vi "Dashboard Main.vi"() -> ()   [LabVIEW 2014]
uses:
  <vilib>/event_ctls.llb/eventvkey.ctl
  <vilib>/Rock Robotics/WPI/Dashboard/WPI_DashboardLogging Global.vi
  <vilib>/Rock Robotics/Network Tables/SD Read Number.vi
  <vilib>/Rock Robotics/Network Tables/SD Write Number.vi
  <vilib>/Utility/config.llb/Write Key (String).vi
  <vilib>/Utility/config.llb/Write Key (I32).vi
  <vilib>/Utility/config.llb/NI_LVConfig.lvlib
panel:
  in  "angle":dbl(slide) scale=0.0..360.0
  in  "kD":dbl
  in  "kI":dbl
  in  "kP":dbl
  out "PID Chart":T1(graph)
  in  "TCP":refnum<k5>
  in  "Rec Mode":enum32{"Stop", "Record", "Playback"}(radio)
  in  "Vision":u16(ring) items=["Camera Off", "USB Camera SW", "USB Camera HW", "IP Camera"]
  out "Camera IP":string
  out "Image Message":string="Timeout in Camera Communications"
  in  "Dashboard Tab":T2(tab)
  in  "Camera Settings":T3={"Frame Rate"=30, "Compression"=30, "Size"=1} {"Frame Rate" scale=1.0..30.0; "Size" items=["640x480", "320x240", "160x120"]}
  out "MotorChart R":cluster{"Numeric":dbl, "Numeric":dbl}(graph)
  out "MotorChart L":T4(graph)
  out "MotorSliders R":cluster{"MotorSlide1":dbl, "MotorSlide2":dbl} {"MotorSlide2" scale=-1.0..1.0 scale format="%#_2e"; "MotorSlide1" scale=-1.0..1.0 scale format="%#_2e"}
  out "MotorSliders L":T5 {"MotorSlide4 2" scale=0.0..14.0 scale format="%#_2e"; "MotorSlide2" scale=-1.0..1.0 scale format="%#_2e"; "MotorSlide1" scale=-1.0..1.0 scale format="%#_2e"}
  out "Gyro":dbl(knob) scale=0.0..360.0
  out "JS1 Z":dbl(slide) scale=-1.0..1.0 scale format="%#_2e"
  out "JS1 Graph":cluster{"X":dbl, "Y":dbl}[](graph)
  out "JS1 Buttons":T6
  out "JS2 Z":dbl(slide) scale=-1.0..1.0 scale format="%#_2e"
  out "JS2 Graph":cluster{"X":dbl, "Y":dbl}[](graph)
  out "JS2 Buttons":T6
  out "Mode":T7(ring)=enum."Auto Disabled"
  in  "DB Camera Config":bool
  out "fps":dbl format="%#.1g"
  out "Mbps":dbl format="%#.1g"
  out "Mbps 2":bool
  in  "DB/String 9":string
  in  "DB/String 8":string
  in  "DB/String 7":string
  in  "DB/String 6":string
  in  "DB/String 5":string
  in  "DB/String 4":string
  in  "DB/String 3":string
  in  "DB/String 2":string
  in  "DB/String 1":string
  in  "DB/String 0":string
  in  "DB/Slider 0":dbl(slide) scale=0.0..5.0
  in  "DB/Slider 1":dbl(slide) scale=0.0..5.0
  in  "DB/Slider 2":dbl(slide) scale=0.0..5.0
  in  "DB/Slider 3":dbl(slide) scale=0.0..5.0
  out "DB/LED 3":bool
  out "DB/LED 2":bool
  out "DB/LED 1":bool
  out "DB/LED 0":bool
  in  "DB/Button 3":bool
  in  "DB/Button 2":bool
  in  "DB/Button 1":bool
  in  "DB/Button 0":bool caption="New Name"
  in  "Test Slider":dbl(slide) scale=0.0..100.0 scale format="%#_3g"
  in  "On/Off":bool caption="Solenoid"
  in  "Test Name":u16(ring) items=["Select the test to run...", "Example Test", "-------------------------------", "List of tests is built in robot code.", "Replace with your own automated tests."]
  in  "Test Tree":string(tree)
  in  "Motor":cluster{"Value":dbl, "Enable":bool} {"Value" scale=-1.0..1.0 scale format="%#_3g"}
  out "Progress":T8 {"Test Progress" scale=0.0..100.0}
  in  "Rev/Fwd":cluster{"Forward":bool, "Reverse":bool}
  in  "Test Ring":u16(ring) items=["Monochrome", "Color"]
  in  "Listbox":i32(listbox)
  out "Tree":string(tree)
  out "Camera Image":T9(plugin-control)
  out "Boolean":bool
  # "Left"
  # "Front"
  # "Right"
  # "Battery"
  # "This tab is a great place for autonomous settings and robot-specific values.\nPlace controls and indicators inside this tab and match name to\nDashboard Variables on robot. You can also delete this comment."
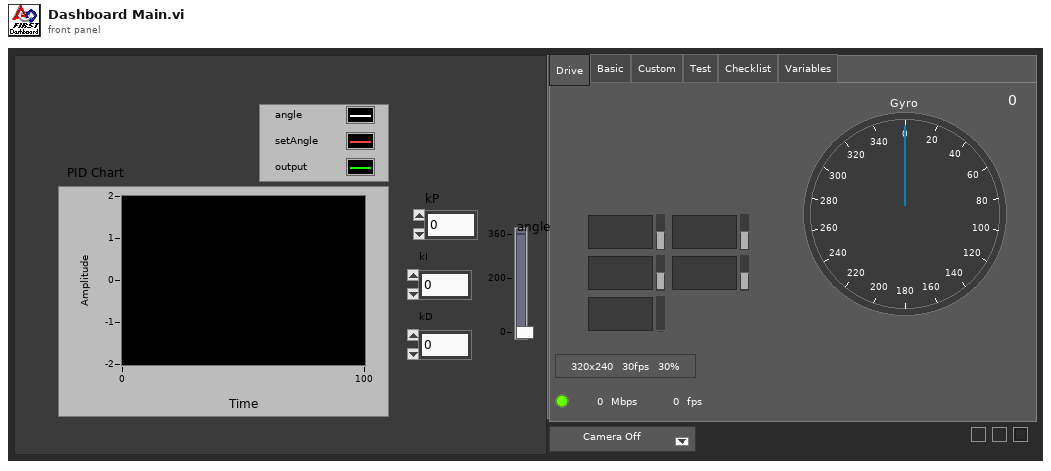
[diagram p1: front panel]
types:
  T1 = cluster{"Numeric":dbl, "Numeric":dbl, "Numeric":dbl}
  T2 = enum32{"Drive", "Basic", "Custom", "Test", "Checklist", "Variables"}
  T3 = cluster{"Frame Rate":i32, "Compression":i32, "Size":u16}
  T4 = cluster{"Numeric":dbl, "Numeric":dbl, "Battery V":dbl}
  T5 = cluster{"MotorSlide1":dbl, "MotorSlide2":dbl, "MotorSlide4 2":dbl}
  T6 = cluster{bool, bool, bool, bool, bool, bool, bool, bool, bool, bool, bool, bool}
  T7 = enum8{"Tele-Op Disabled", "Tele-Op Enabled", "Auto Disabled", "Auto Enabled", "Test Disabled", "Test Enabled", "Disconnected", "No Code", "E-Stop"}
  T8 = cluster{"Test Progress":u8, "Test Progress Text":string}
  T9 = typedef "IMAQ Image.ctl" = refnum<image>
  T10 = typedef "Image Type" = u32
  T11 = cluster{"Camera Image":refnum<vi>, "Dashboard Tab":refnum<vi>, "Boolean":refnum<vi>, "Vision":refnum<vi>, "Rec Mode":refnum<vi>, "Test Slider":refnum<vi>, "On/Off ":refnum<vi>, "Test Ring":refnum<vi>, "Rev/Fwd":refnum<vi>, "Test Name":refnum<vi>, "Motor":refnum<vi>, "Progress":refnum<vi>, "CheckList":refnum<vi>, "Tree":refnum<vi>, "Test Tree":refnum<vi>}
  T12 = cluster{"Error Strings":string, "Disable Counts":cluster{u16, u16}, "Rail Faults":cluster{u16, u16, u16}, "Robot IP":string, "DB Mode":u8, "Event Info":cluster{"Name":string, "Type":u8, "Number":u16, "Replay":u8}, "Camera Addr":string}
  T13 = cluster{"Storage":cluster{"Disk Free":u64, "RAM Block":u32, "RAM free":u32}, "CPU Utilization":cluster{"CPU % ISR":sgl, "CPU % Time Crit":sgl, "CPU % Timed Str":sgl, "CPU % High":sgl, "CPU % Above":sgl, "CPU % Normal":sgl, "CPU % Low":sgl}, "CAN":cluster{"% Bus Utilization":sgl, "Bus Off Cnt":u32, "TX_FIFO Full Cnt":u32, "Receive Error Cnt":u8, "Transmit Error Cnt":u8}, "HID":cluster{"HID Outputs":u32, "Rumble Low":u16, "Rumble High":u16}[]}
  T14 = cluster{"Status bits":cluster{"Test Mode":bool, "Autonomous":bool, "Enabled":bool, "Code Start":bool, "Brownout":bool, "Reserved 2":bool, "Reserved 3":bool, "E-Stop":bool}, "Code Trace":cluster{"Disabled":bool, "TeleOp":bool, "Auto":bool, "Test":bool}, "Controller Type":enum16{"unknown", "cRIO", "roboRio"}, "Code?":enum16{"unknown", "noCode", "code"}, "Battery V":dbl}
  T15 = cluster{"Control Bits":cluster{"TestMode":bool, "Autonomous":bool, "Enabled":bool, "FMS Present":bool, bool, bool, bool, "E-Stop":bool}, "Team Station ":u8, "Countdown":sgl, "Joystick Values":cluster{"Axes":dbl[], "Buttons":bool[], "POVs":i16[]}[]}
  T16 = cluster{"Axes":dbl[], "Buttons":bool[], "POVs":i16[]}[]
  T17 = cluster{"Axes":dbl[], "Buttons":bool[], "POVs":i16[]}
  T18 = cluster{"Buttons[0]":bool, "Buttons[1]":bool, "Buttons[2]":bool, "Buttons[3]":bool, "Buttons[4]":bool, "Buttons[5]":bool, "Buttons[6]":bool, "Buttons[7]":bool, "Buttons[8]":bool, "Buttons[9]":bool, "Buttons[10]":bool, "Buttons[11]":bool}
  T19 = typedef "NI_LVConfig.lvlib/Config Data RefNum.ctl" = refnum<k1>
  T20 = cluster{"Operation":enum16{"Update", "Clear"}, "Color Box":u32}[]
  T21 = typedef "eventvkey.ctl" = enum16{"ASCII", "Enter", "Return", "Shift", "Ctrl", "Alt", "Cmd", "Opt", "Caps", "NumLock", "Clear", "Break", "Up", "Down", "Left", "Right", "Insert", "Delete", "Home", "End", "PageUp", "PageDown", "Escape", "Help", "Pause", "ScrollLock", "F1", "F2", "F3", "F4", "F5", "F6", "F7", "F8", "F9", "F10", "F11", "F12", "F13", "F14", "F15", "F16", "F17", "F18", "F19", "F20", "F21", "F22", "F23", "F24", "Play", "VolumeUp", "VolumeDown", "Mute", "Two Byte Char"}
  T22 = cluster{"Image Size":bool, "Image Type":bool, "Pixel Value":bool, "ROI Information":bool, "Zoom Factor":bool}
  T23 = enum8{"Enabled", "Disabled", "Disabled and Grayed Out"}
  T24 = cluster{"Operation":enum16{"Update", "Clear"}, "Color Box":u32}
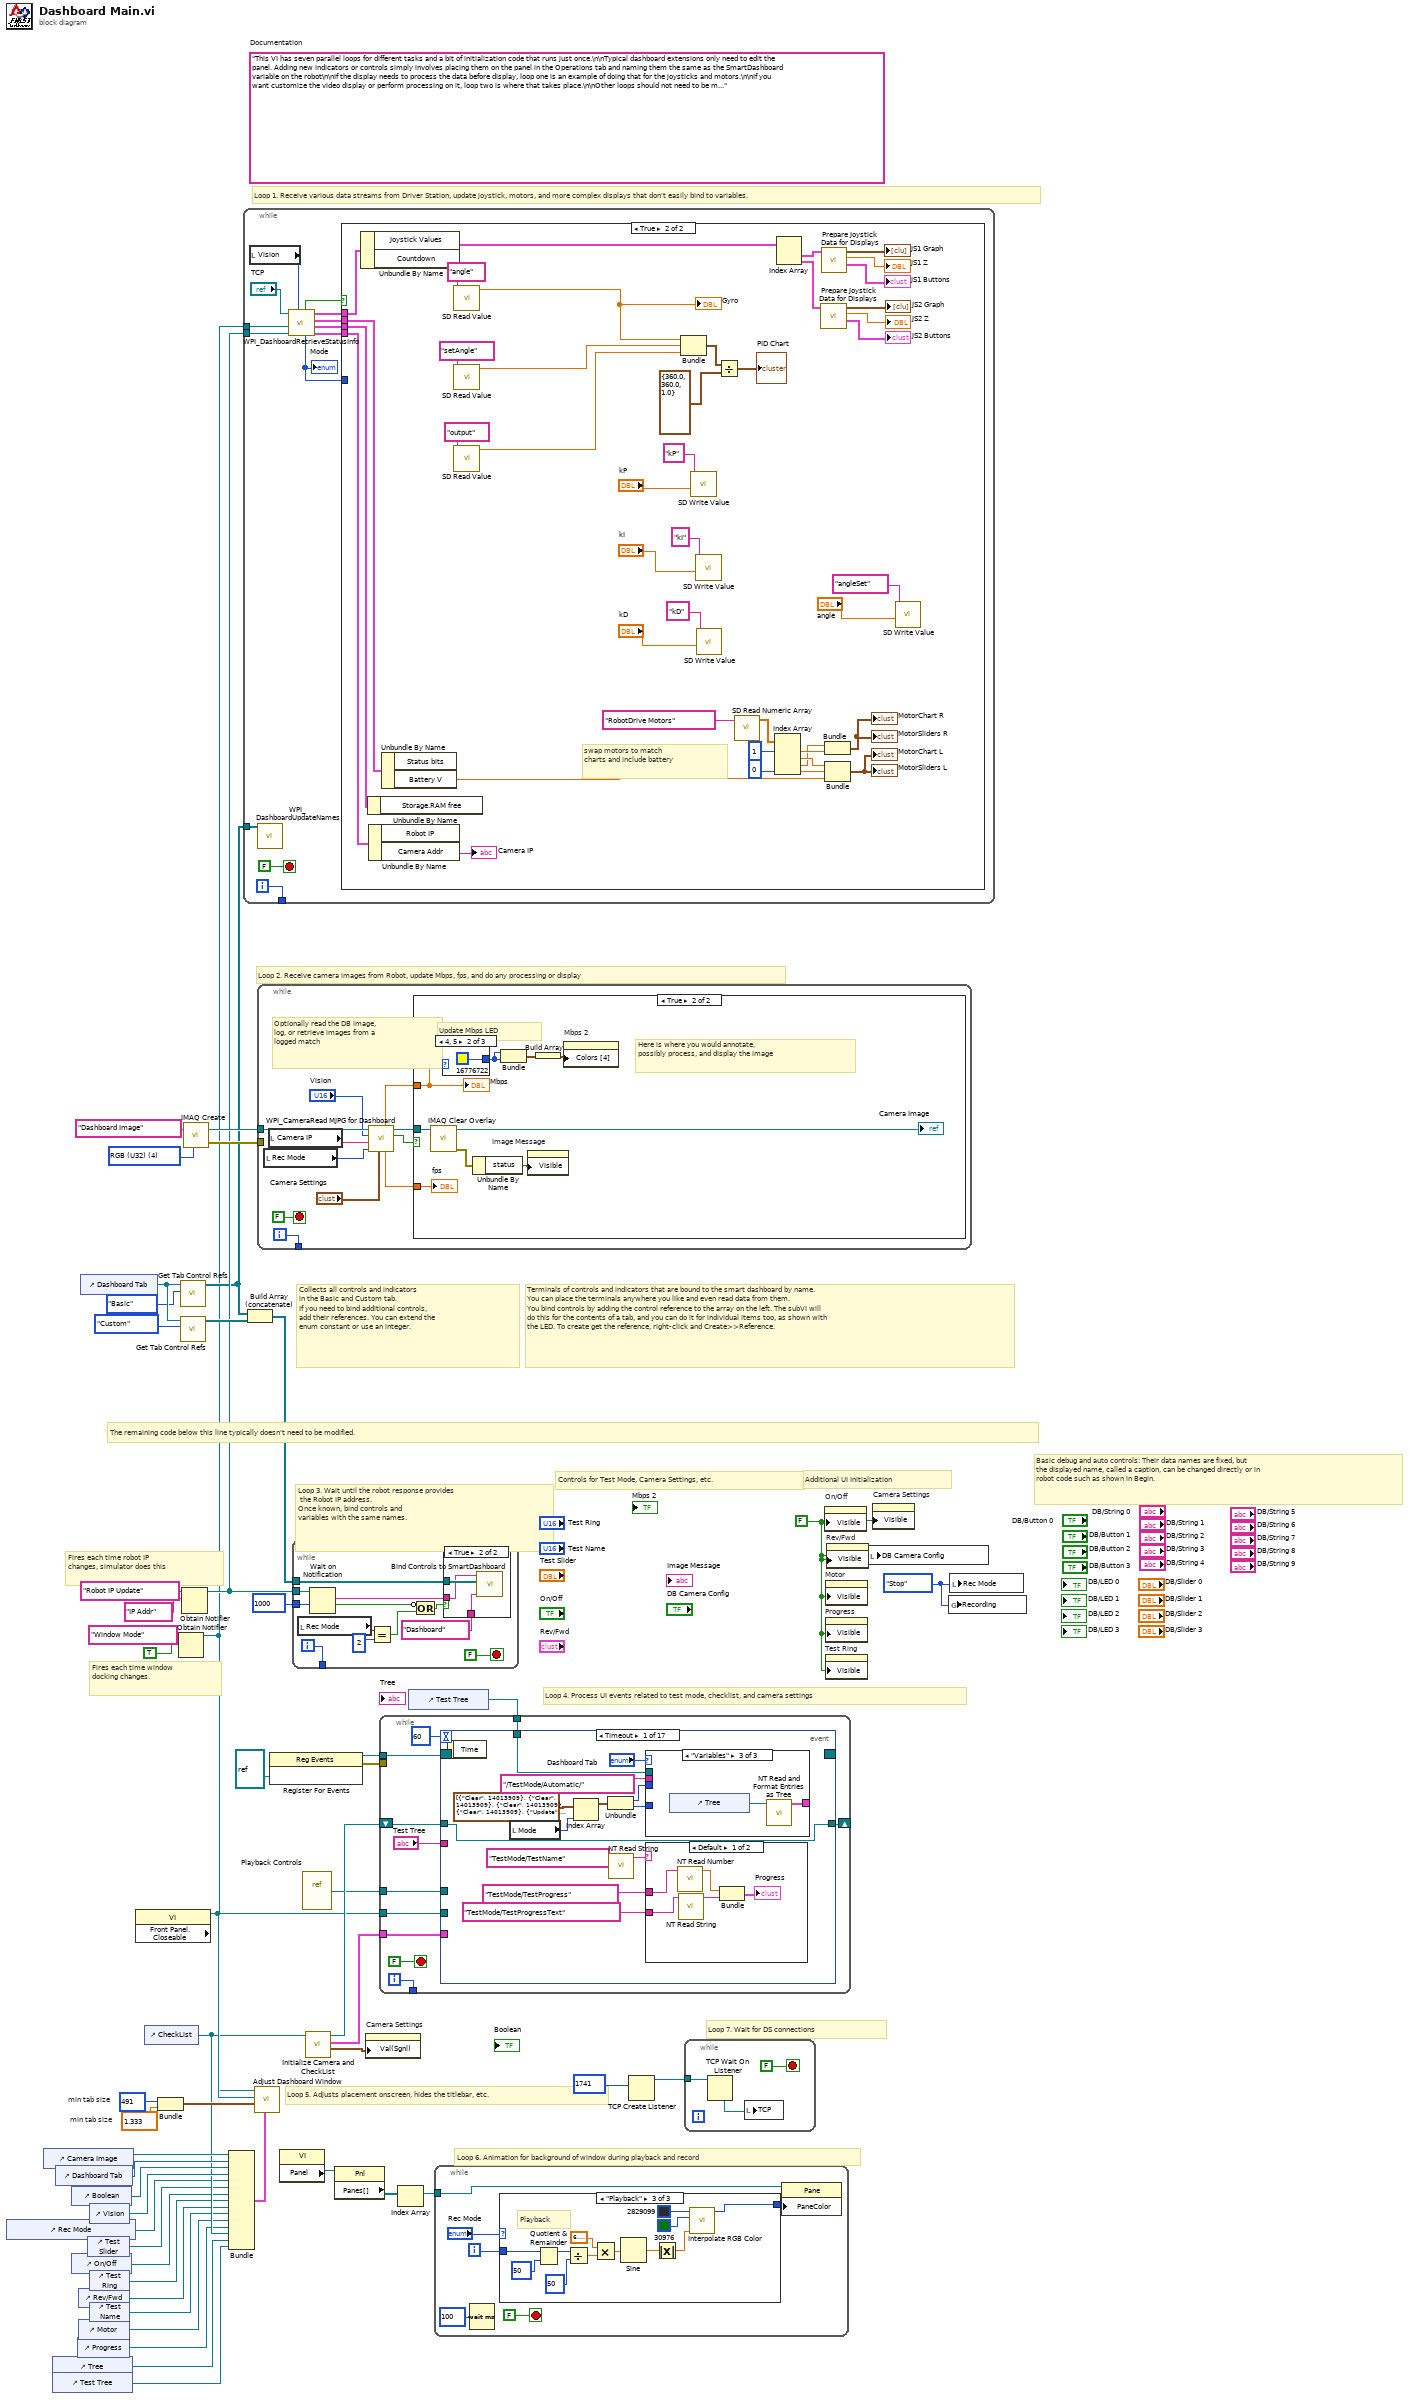
[diagram p0: block diagram]
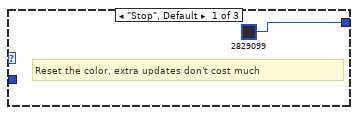
[diagram p3: hidden frame]
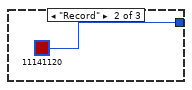
[diagram p4: hidden frame]
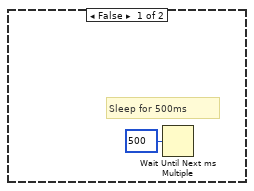
[diagram p6: hidden frame]
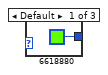
[diagram p7: hidden frame]
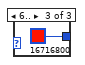
[diagram p8: hidden frame]
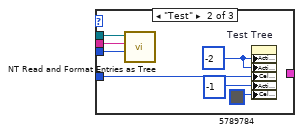
[diagram p10: hidden frame]
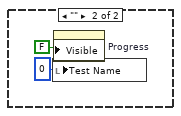
[diagram p11: hidden frame]
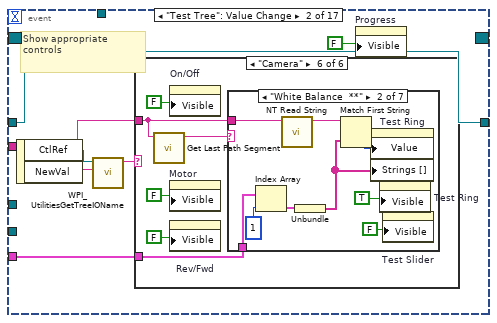
[diagram p12: hidden frame]
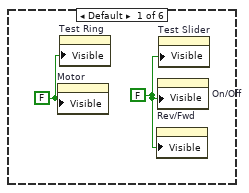
[diagram p13: hidden frame]
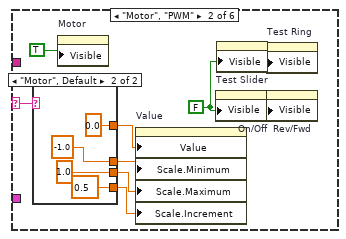
[diagram p14: hidden frame]
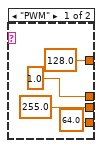
[diagram p15: hidden frame]
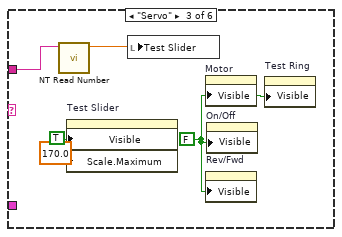
[diagram p16: hidden frame]
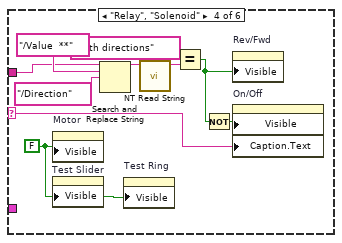
[diagram p17: hidden frame]
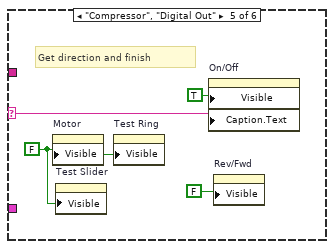
[diagram p18: hidden frame]
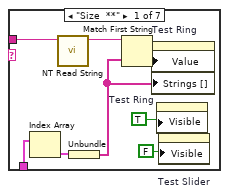
[diagram p19: hidden frame]
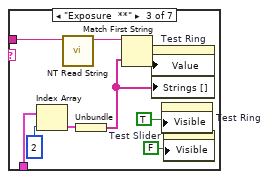
[diagram p20: hidden frame]
diagram:
  w24 = 491  # min tab size
  w23 = 1.333  # min tab size
  w32 = enum32{"Stop", "Record", "Playback"}."Stop" ("Rec Mode")
  w6 = FALSE ("Visible")
  (unwired) "This VI has seven parallel loops for different tasks and a bit of initialization code that runs just once.\n\nTypical dashboard extensions only need to edit the panel. Adding new indicators or controls simply involves placing them on the panel in the Operations tab and naming them the same as the SmartDashboard variable on the robot\n\nIf the display needs to process the data before display, loop one is an example of doing that for the joysticks and motors.\n\nIf you want customize the video display or perform processing on it, loop two is where that takes place.\n\nOther loops should not need to be modified. They are pretty standard, and document the task they perform."  # Documentation
  w52 = T10 4 items=["Grayscale (U8)", "Grayscale (I16)", "Grayscale (SGL)", "Complex (CSG)", "RGB (U32)", "HSL (U32)", "RGB (U64)"] ("Image Type")
  # "Loop 7. Wait for DS connections"
  # "Basic debug and auto controls: Their data names are fixed, but\nthe displayed name, called a caption, can be changed directly or in\nrobot code such as shown in Begin."
  # "Controls for Test Mode, Camera Settings, etc."
  # "Additional UI Initialization"
  # "Loop 6. Animation for background of window during playback and record"
  # "Fires each time robot IP\nchanges, simulator does this"
  # "Fires each time window\ndocking changes."
  # "Collects all controls and indicators\nin the Basic and Custom tab.\nIf you need to bind additional controls,\nadd their references. You can extend the\nenum constant or use an integer."
  # "The remaining code below this line typically doesn't need to be modified."
  # "Loop 4. Process UI events related to test mode, checklist, and camera settings"
  # "Terminals of controls and indicators that are bound to the smart dashboard by name.\nYou can place the terminals anywhere you like and even read data from them.\nYou bind controls by adding the control reference to the array on the left. The subVI will\ndo this for the contents of a tab, and you can do it for individual items too, as shown with\nthe LED. To create get the reference, right-click and Create>>Reference."
  # "Loop 3. Wait until the robot response provides\n the Robot IP address.\nOnce known, bind controls and\nvariables with the same names."
  # "Loop 5. Adjusts placement onscreen, hides the titlebar, etc."
  # "Loop 1. Receive various data streams from Driver Station, update joystick, motors, and more complex displays that don't easily bind to variables."
  # "Loop 2. Receive camera images from Robot, update Mbps, fps, and do any processing or display"
  n1 = control-ref of="Rec Mode"() -> (w12:refnum<vi>)
  n2 = control-ref of="Camera Image"() -> (w27:refnum<vi>)
  n3 = control-ref of="Tree"() -> (w16:refnum<vi>)
  n4 = control-ref of="Test Tree"() -> (w15:refnum<vi>)
  n5 = control-ref of="Dashboard Tab"() -> (w26:refnum<vi>)
  n6 = control-ref of="Boolean"() -> (w21:refnum<vi>)
  n7 = control-ref of="On/Off"() -> (w10:refnum<vi>)
  n8 = control-ref of="Progress"() -> (w7:refnum<vi>)
  n9 = control-ref of="Rev/Fwd"() -> (w8:refnum<vi>)
  n10 = control-ref of="Motor"() -> (w13:refnum<vi>)
  n11 = control-ref of="Dashboard Tab"() -> (w30:refnum<vi>)
  n12 = control-ref of="Test Slider"() -> (w11:refnum<vi>)
  n13 = control-ref of="Vision"() -> (w25:refnum<vi>)
  n14 = control-ref of="Test Ring"() -> (w9:refnum<vi>)
  n15 = control-ref of="Test Name"() -> (w14:refnum<vi>)
  n16 = property class="VI" props=["Front Panel.Closeable"]() -> (reference out=w31:refnum<vi>)  [unwired: 2 in, 2 out]
  n17 = control-ref of="CheckList"() -> (w17:refnum<vi>)
  n18 = Bundle("min tab size"=w24, "min tab size"=w23) -> (w22:cluster{"min tab size":i32, "min tab size":dbl})  [unwired: 1 in]
  n19 = Obtain Notifier(name (unnamed)="Window Mode", notification data type=TRUE) -> (notifier out=w3:refnum<notifier>)  [unwired: 2 in, 2 out]
  n20 = call <vilib>:"Get Tab Control Refs.vi"("Page Index"=T2."Basic" ("Dashboard Tab"), "TabControl in"=w30) -> ("ControlsOnPage"=w4:refnum<vi>[])  [unwired: 9 in]
  n21 = call <vilib>:"Get Tab Control Refs.vi"("Page Index"=T2."Custom" ("Dashboard Tab"), "TabControl in"=w30) -> ("ControlsOnPage"=w29:refnum<vi>[])  [unwired: 9 in]
  n22 = Obtain Notifier(name (unnamed)="Robot IP Update", notification data type="IP Addr" ("name (unnamed)")) -> (notifier out=w5:refnum<notifier>)  [unwired: 2 in, 2 out]
  n23 = call "IMAQ Create"("Image Name"="Dashboard Image", "Image Type"=w52) -> ("New Image"=w50:T9, "error out"=w49:errorcluster)  [unwired: 2 in, 1 out]
  n24 = Bundle("Camera Image"=w27, "Dashboard Tab"=w26, "Boolean"=w21, "Vision"=w25, "Rec Mode"=w12, "Test Slider"=w11, "On/Off"=w10, "Test Ring"=w9, "Rev/Fwd"=w8, "Test Name"=w14, "Motor"=w13, "Progress"=w7, "CheckList"=w17, "Tree"=w16, "Test Tree"=w15) -> (w18:T11)  [unwired: 1 in]
  n25 = while {
    tunnel: [w64] -> _
    tunnel: w5 -> [w58]
    tunnel: w4 -> [w57]
    tunnel: w3 -> [w53]
    i -> [w64]
    stop <- FALSE stop-if-true
    n26 = local read "Vision"() -> (w55:u16)
    n27 = call <vilib>:"WPI_DashboardUpdateNames.vi"("Controls on Tab"=w57) -> ()  [unwired: 11 in]
    n28 = call <vilib>:"WPI_DashboardRetrieveStatusInfo.vi"("Vision"=w55, "Binding Refnum"=w58, "Window Mode Notifier"=w53, "TCP Cnx"="TCP") -> ("Power and Errors"=w59:T12, "Robot Metrics"=w62:T13, "Status Info"=w63:T14, "Control Info"=w60:T15, "Robot Mode"=w56:T7, "Process?"=w61:bool)  [unwired: 2 in]
    "Mode" <- w56
    n29 = case shown="True" w61 {
      tunnel: w63 -> [_ w107]
      tunnel: w62 -> [_ w106]
      tunnel: w60 -> [_ w105]
      tunnel: w59 -> [_ w104]
      tunnel: w56 -> [_ _]
      frame False {
      }
      frame True {
        # "swap motors to match\ncharts and include battery"
        n30 = Unbundle By Name(w105) -> ("Joystick Values"=w92:T16)  [unwired: 1 out]
        n31 = Unbundle By Name(w106) -> ()  [unwired: 1 out]
        n32 = Unbundle By Name(w104) -> ("Camera Addr"=→"Camera IP":string)  [unwired: 1 out]
        n33 = Unbundle By Name(w107) -> ("Battery V"=w93:dbl)  [unwired: 1 out]
        n34 = call-poly <vilib>:"SD Read Value.vi"("Name"="angle") -> ("Numeric"=w68:dbl)  [unwired: 8 in, 2 out]
        "Gyro" <- w68
        n35 = call-poly <vilib>:"SD Read Value.vi"("Name"="setAngle") -> ("Numeric"=w80:dbl)  [unwired: 8 in, 2 out]
        n36 = call-poly <vilib>:"SD Read Value.vi"("Name"="output") -> ("Numeric"=w78:dbl)  [unwired: 8 in, 2 out]
        n37 = Bundle("Numeric"=w68, "Numeric"=w80, "Numeric"=w78) -> (w76:T1)  [unwired: 1 in]
        n38 = call-poly <vilib>:"SD Write Value.vi"("Numeric"="kP", "Name"="kP") -> ()  [unwired: 8 in, 2 out]
        n39 = call-poly <vilib>:"SD Write Value.vi"("Numeric"="kI", "Name"="kI") -> ()  [unwired: 8 in, 2 out]
        n40 = call-poly <vilib>:"SD Write Value.vi"("Numeric"="kD", "Name"="kD") -> ()  [unwired: 8 in, 2 out]
        n41 = Divide(x=w76, y=T1 {"Numeric"=360.0, "Numeric"=360.0, "Numeric"=1.0}) -> (x/y=→"PID Chart":T1)
        n42 = call <vilib>:"SD Read Numeric Array.vi"("Name"="RobotDrive Motors") -> ("Numeric Array"=w95:dbl[])  [unwired: 8 in, 2 out]
        n43 = Index Array(array=w95, index #1=1, index #4=0) -> (element #1=w99:dbl, element #2=w100:dbl, element #3=w98:dbl, element #4=w103:dbl)  [unwired: 2 in]
        n44 = Index Array(array=w92) -> (element #1=w91:T17, element #2=w86:T17)  [unwired: 2 in]
        n45 = call "Prepare Joystick Data for Displays.vi"("Joystick Values"=w86) -> ("Buttons"=→"JS2 Buttons":T18, "Z Axis"=→"JS2 Z":dbl, "Cartesian Data"=→"JS2 Graph":cluster{"X axis":dbl, "X axis":dbl}[])  [unwired: 8 in]
        n46 = call "Prepare Joystick Data for Displays.vi"("Joystick Values"=w91) -> ("Buttons"=→"JS1 Buttons":T18, "Z Axis"=→"JS1 Z":dbl, "Cartesian Data"=→"JS1 Graph":cluster{"X axis":dbl, "X axis":dbl}[])  [unwired: 8 in]
        n47 = Bundle("Numeric"=w98, "Numeric"=w99) -> (→"MotorChart R" →"MotorSliders R":cluster{"Numeric":dbl, "Numeric":dbl})  [unwired: 1 in]
        n48 = Bundle("Numeric"=w100, "Numeric"=w103, "Battery V"=w93) -> (→"MotorChart L" →"MotorSliders L":T4)  [unwired: 1 in]
        n49 = call-poly <vilib>:"SD Write Value.vi"("Numeric"="angle", "Name"="angleSet") -> ()  [unwired: 8 in, 2 out]
      }
    }
  }
  n50 = Build Array (concatenate)(w4, w29) -> (w28:refnum<vi>[])
  n51 = call "Adjust Dashboard Window.vi"("Sizing Refnums"=w18, "Size Constraints"=w22, "VI"=w31, "Notifier in"=w3) -> ()  [unwired: 8 in]
  n52 = while {
    tunnel: w50 -> [w116]
    tunnel: w49 -> [_]
    tunnel: [w117] -> _
    i -> [w117]
    stop <- FALSE stop-if-true
    # "Optionally read the DB image,\nlog, or retrieve images from a\nlogged match"
    n53 = local read "Rec Mode"() -> (w110:enum32{"Stop", "Record", "Playback"})
    n54 = local read "Camera IP"() -> (w108:string)
    n55 = call <vilib>:"WPI_CameraRead MJPG for Dashboard.vi"("Camera Settings"="Camera Settings", "Rec Mode"=w110, "Camera IP"=w108, "Camera Mode"="Vision", "Refnum in"=w116) -> ("Active"=w114:bool, "Refnum out"=w115:T9, "FPS"=w113:dbl, "Bandwidth (Mbps)"=w112:dbl)  [unwired: 3 in]
    n56 = case shown="True" w114 {
      tunnel: w115 -> [_ w123]
      tunnel: w112 -> [_ w122]
      tunnel: w113 -> [_ w120]
      frame False {
        # "Sleep for 500ms"
        n57 = Wait Until Next ms Multiple(millisecond multiple=u32 500) -> ()  [unwired: 1 out]
      }
      frame True {
        # "Here is where you would annotate,\npossibly process, and display the image"
        # "Update Mbps LED"
        n58 = call "IMAQ Clear Overlay"("Image"=w123) -> ("error out"=w127:errorcluster, "Image Out"=→"Camera Image":T9)  [unwired: 2 in, 7 out]
        n59 = case shown="4, 5" w122 {
          tunnel: [u32 6618880 ("Color Box") u32 16776722 ("Color Box") u32 16716800 ("Color Box")] -> w124
          frame Default {
          }
          frame 4, 5 {
          }
          frame 6.. {
          }
        }
        n60 = Unbundle By Name(w127) -> ("status"=w128:bool)
        n61 = Bundle("Color Box"=w124, "Color Box"=w124) -> (w126:cluster{"Color Box":u32, "Color Box":u32})  [unwired: 1 out]
        n62 = property on="Image Message" class="Str"("Visible"=w128) -> ()  [unwired: 2 in, 2 out]
        n63 = Build Array(w126) -> (w125:cluster{"Color Box":u32, "Color Box":u32}[])
        n64 = property on="Mbps 2" class="Bool (strict)"("Colors [4]"=w125) -> ()  [unwired: 2 in, 2 out]
        "Mbps" <- w122
        "fps" <- w120
      }
    }
  }
  n65 = register-events(refnum<vi> refnum) -> (reference out=w36:refnum<event-registration>, error out=w35:errorcluster)  [unwired: 2 in]
  n66 = property class="VI"() -> ("Panel"=w39:refnum<vi>)  [unwired: 2 in, 2 out]
  n67 = while {
    tunnel: w28 -> [w143]
    tunnel: w5 -> [w141]
    tunnel: [w139] -> _
    tunnel: u32 1000 ("milliseconds to wait") -> [w138]
    i -> [w139]
    stop <- FALSE stop-if-true
    n68 = local read "Rec Mode"() -> (w134:enum32{"Stop", "Record", "Playback"})
    n69 = Wait on Notification(notifier=w141, timeout in ms (-1)=w138) -> (notification=w140:string, timed out?=w136:bool)  [unwired: 2 in, 2 out]
    n70 = Equal?(x=w134, y=u16 2 ("Rec Mode")) -> (x = y?=w135:bool)
    n71 = Compound Arithmetic op=OR(invert w136, w135) -> (w137:bool)
    n72 = case shown="True" w137 {
      tunnel: w143 -> [_ w146]
      tunnel: w140 -> [_ w145]
      tunnel: "Dashboard" -> [_ w144]
      frame False {
      }
      frame True {
        n73 = call <vilib>:"Bind Controls to SmartDashboard.vi"("Client Name"=w144, "Bound Control Refs"=w146, "Server IP Address"=w145) -> ()  [unwired: 9 in]
      }
    }
  }
  n74 = vi-ref "Playback Controls.vi"() -> (w37:refnum<vi>)
  n75 = call "Initialize Camera and CheckList.vi"("ListBox in"=w17) -> ("Cluster"=w43:cluster{"value":i32, "value":i32, "index":i32}, "Array"=w44:cluster{string[]}[], "File Refnum"=w42:T19)  [unwired: 8 in]
  n76 = property class="Pnl"(reference=w39) -> ("Panes[]"=w40:refnum<vi>[])  [unwired: 1 in, 2 out]
  n77 = property on="Camera Settings" class="Clust (strict)"("Val(Sgnl)"=w43) -> ()  [unwired: 2 in, 2 out]
  n78 = Index Array(array=w40) -> (element=w38:refnum<vi>)  [unwired: 1 in]
  n79 = control-ref of="Test Tree"() -> (w41:refnum<vi>)
  n80 = while {
    tunnel: w44 -> [w154]
    shift-right: [w153] -> _
    shift-left: w42 -> [w152]
    tunnel: [w151] -> _
    tunnel: w41 -> [w150]
    tunnel: w37 -> [w149]
    tunnel: w36 -> [w148]
    tunnel: w35 -> [_]
    tunnel: w31 -> [w147]
    i -> [w151]
    stop <- FALSE stop-if-true
    n81 = event shown="[0] Timeout" {
      selector: w148 -> [_ _ _ _ _ _ _ _ _ _ _ _ _ _ _ _ _]
      dyn-events: [_ _ _ _ _ _ _ _ _ _ _ _ _ w392 _ _ _] -> _
      timeout: u32 60 ("milliseconds to wait") -> [_ _ _ _ _ _ _ _ _ _ _ _ _ _ _ _ _]
      tunnel: w150 -> [w166 _ _ _ _ _ _ _ _ _ _ _ _ _ _ _ _]
      tunnel: "Test Tree" -> [_ _ _ _ _ _ _ _ w361 w369 w371 w375 w383 _ _ _ _]
      tunnel: w154 -> [_ w188 _ _ _ _ w325 w355 _ _ _ _ _ _ _ _ _]
      tunnel: [w162 w187 w286 w291 w299 w311 w324 w348 w360 w367 w370 w374 w382 w394 w408 w409 w419] -> w153
      tunnel: w152 -> [w162 w187 w286 w291 w299 w311 w323 w348 w360 w367 w370 w374 w382 w394 w408 w409 w419]
      tunnel: w149 -> [_ _ _ _ _ _ _ _ _ _ _ _ _ w395 _ w412 _]
      tunnel: w147 -> [_ _ _ _ _ _ _ _ _ _ _ _ _ w390 _ _ _]
      event Timeout {
        n82 = event-data() -> ()  [unwired: 1 in, 1 out]
        n83 = local read "Mode"() -> (w165:T7)
        n84 = Index Array(array=T20 [{"Operation"=enum."Clear", "Color Box"=14013909}, {"Operation"=enum."Clear", "Color Box"=14013909}, {"Operation"=enum."Clear", "Color Box"=14013909}, {"Operation"=enum."Clear", "Color Box"=14013909}, {"Operation"=enum."Update", "Color Box"=14013909}, {"Operation"=enum."Update", "Color Box"=16777215}, {"Operation"=enum."Clear", "Color Box"=14013909}, {"Operation"=enum."Clear", "Color Box"=14013909}, {"Operation"=enum."Clear", "Color Box"=14013909}], index=w165) -> (element=w160:T24)
        n85 = Unbundle(w160) -> ("Operation"=w159:enum16{"Update", "Clear"}, "Color Box"=w158:u32)
        n86 = call <vilib>:"NT Read String.vi"("Name"="TestMode/TestName") -> ("String"=w169:string)  [unwired: 9 in, 1 out]
        n87 = case shown="\"Variables\"" "Dashboard Tab" {
          tunnel: w166 -> [_ w177 _]
          tunnel: "/TestMode/Automatic/" ("Name Pattern") -> [_ w176 _]
          tunnel: w159 -> [_ w175 _]
          tunnel: [_ _ w179] -> _
          tunnel: w158 -> [_ w171 _]
          frame "Custom", Default {
          }
          frame "Test" {
            w174 = -2 ("Active Item:Row Number")
            n88 = call <vilib>:"NT Read and Format Entries as Tree.vi"("Operation"=w175, "Name Pattern"=w176, "Tree Refnum"=w177) -> ()  [unwired: 7 in, 2 out]
            n89 = property on="Test Tree" class="Tree (strict)"("Active Item Row Number"=w174, "ActiveColNum"=w174, "CellBG"=w171, "Active Item Row Number"=-1 ("Active Item:Row Number"), "CellBG"=u32 5789784 ("Color Box")) -> ()  [unwired: 2 in, 2 out]
          }
          frame "Variables" {
            n90 = control-ref of="Tree"() -> (w178:refnum<vi>)
            n91 = call <vilib>:"NT Read and Format Entries as Tree.vi"("Tree Refnum"=w178) -> ("Formatted Strings"=w179:cluster{"Name":string, "Value":string}[])  [unwired: 9 in, 1 out]
          }
        }
        n92 = case shown="Default" w169 {
          tunnel: "TestMode/TestProgress" ("Name") -> [w181 _]
          tunnel: "TestMode/TestProgressText" ("Name") -> [w180 _]
          frame Default {
            n93 = call <vilib>:"NT Read Number.vi"("Name"=w181) -> ("Numeric"=w182:dbl)  [unwired: 9 in, 1 out]
            n94 = call <vilib>:"NT Read String.vi"("Name"=w180) -> ("String"=w183:string)  [unwired: 9 in, 1 out]
            n95 = Bundle("Numeric"=w182, "String"=w183) -> (→"Progress":cluster{"Numeric":dbl, "String":string})  [unwired: 1 in]
          }
          frame "" {
            n96 = local write "Test Name"(u16 0) -> ()
            n97 = property on="Progress" class="Clust (strict)"("Visible"=FALSE) -> ()  [unwired: 2 in, 2 out]
          }
        }
      }
      event "Test Tree": Value Change {
        # "Show appropriate\ncontrols"
        n98 = event-data() -> ("CtlRef"=w191:refnum<vi>, "NewVal"=w189:string)  [unwired: 1 in]
        n99 = call <vilib>:"WPI_UtilitiesGetTreeIOName.vi"("NewVal"=w189, "TreeControl in"=w191) -> ("I/O Name"=w192:string)  [unwired: 9 in]
        n100 = case shown="\"Camera\"" w192 {
          selector: w192 -> [_ w199 _ w217 w226 _]
          tunnel: w189 -> [_ _ w214 w216 _ w233]
          tunnel: w188 -> [_ _ _ _ _ w232]
          frame Default {
            w194 = FALSE ("Visible")
            w193 = FALSE ("Visible")
            n101 = property on="Motor" class="Clust (strict)"("Visible"=w193) -> ()  [unwired: 2 in, 2 out]
            n102 = property on="Test Ring" class="Ring (strict)"("Visible"=w193) -> ()  [unwired: 2 in, 2 out]
            n103 = property on="Rev/Fwd" class="Clust (strict)"("Visible"=w194) -> ()  [unwired: 2 in, 2 out]
            n104 = property on="On/Off" class="Bool (strict)"("Visible"=w194) -> ()  [unwired: 2 in, 2 out]
            n105 = property on="Test Slider" class="Slide (strict)"("Visible"=w194) -> ()  [unwired: 2 in, 2 out]
          }
          frame "Motor", "PWM" {
            w200 = FALSE ("Visible")
            n106 = case shown="\"Motor\", Default" w199 {
              tunnel: [1.0 ("Value") -1.0 ("Value")] -> w198
              tunnel: [255.0 ("Value") 1.0 ("Value")] -> w197
              tunnel: [128.0 ("Value") 0.0 ("Value")] -> w196
              tunnel: [64.0 ("Value") 0.5 ("Value")] -> w195
              frame "PWM" {
              }
              frame "Motor", Default {
              }
            }
            n107 = property on="Motor" class="Clust (strict)"("Visible"=TRUE) -> ()  [unwired: 2 in, 2 out]
            n108 = property on="Value" class="Slide (strict)"("Value"=w196, "Scale.Minimum"=w198, "Scale.Maximum"=w197, "Scale.Increment"=w195) -> ()  [unwired: 2 in, 2 out]
            n109 = property on="On/Off" class="Bool (strict)"("Visible"=w200) -> ()  [unwired: 2 in, 2 out]
            n110 = property on="Test Slider" class="Slide (strict)"("Visible"=w200) -> ()  [unwired: 2 in, 2 out]
            n111 = property on="Test Ring" class="Ring (strict)"("Visible"=w200) -> ()  [unwired: 2 in, 2 out]
            n112 = property on="Rev/Fwd" class="Clust (strict)"("Visible"=w200) -> ()  [unwired: 2 in, 2 out]
          }
          frame "Servo" {
            w212 = FALSE ("Visible")
            n113 = call <vilib>:"NT Read Number.vi"("Name"=w214) -> ("Numeric"=w213:dbl)  [unwired: 9 in, 1 out]
            n114 = property on="Test Slider" class="Slide (strict)"("Visible"=TRUE, "Scale.Maximum"=170.0 ("Scale.Range:Maximum")) -> ()  [unwired: 2 in, 2 out]
            n115 = local write "Test Slider"(w213) -> ()
            n116 = property on="Motor" class="Clust (strict)"("Visible"=w212) -> ()  [unwired: 2 in, 2 out]
            n117 = property on="Rev/Fwd" class="Clust (strict)"("Visible"=w212) -> ()  [unwired: 2 in, 2 out]
            n118 = property on="On/Off" class="Bool (strict)"("Visible"=w212) -> ()  [unwired: 2 in, 2 out]
            n119 = property on="Test Ring" class="Ring (strict)"("Visible"=w212) -> ()  [unwired: 2 in, 2 out]
          }
          frame "Relay", "Solenoid" {
            w215 = FALSE ("Visible")
            n120 = property on="Motor" class="Clust (strict)"("Visible"=w215) -> ()  [unwired: 2 in, 2 out]
            n121 = property on="Test Slider" class="Slide (strict)"("Visible"=w215) -> ()  [unwired: 2 in, 2 out]
            n122 = Search and Replace String(input string=w216, search string="/Value  **", replace string="/Direction") -> (result string=w222:string)  [unwired: 5 in, 3 out]
            n123 = property on="Test Ring" class="Ring (strict)"("Visible"=w215) -> ()  [unwired: 2 in, 2 out]
            n124 = call <vilib>:"NT Read String.vi"("Name"=w222) -> ("String"=w220:string)  [unwired: 9 in, 1 out]
            n125 = Equal?(x="Both directions", y=w220) -> (x = y?=w218:bool)
            n126 = Not(x=w218) -> (.not. x?=w219:bool)
            n127 = property on="Rev/Fwd" class="Clust (strict)"("Visible"=w218) -> ()  [unwired: 2 in, 2 out]
            n128 = property on="On/Off" class="Bool (strict)"("Visible"=w219, "Caption.Text"=w217) -> ()  [unwired: 2 in, 2 out]
          }
          frame "Compressor", "Digital Out" {
            w225 = FALSE ("Visible")
            # "Get direction and finish"
            n129 = property on="Motor" class="Clust (strict)"("Visible"=w225) -> ()  [unwired: 2 in, 2 out]
            n130 = property on="Test Slider" class="Slide (strict)"("Visible"=w225) -> ()  [unwired: 2 in, 2 out]
            n131 = property on="Test Ring" class="Ring (strict)"("Visible"=w225) -> ()  [unwired: 2 in, 2 out]
            n132 = property on="On/Off" class="Bool (strict)"("Visible"=TRUE, "Caption.Text"=w226) -> ()  [unwired: 2 in, 2 out]
            n133 = property on="Rev/Fwd" class="Clust (strict)"("Visible"=FALSE) -> ()  [unwired: 2 in, 2 out]
          }
          frame "Camera" {
            n134 = call <vilib>:"Get Last Path Segment.vi"("String in"=w233) -> ("String out"=w234:string)  [unwired: 10 in]
            n135 = property on="On/Off" class="Bool (strict)"("Visible"=FALSE) -> ()  [unwired: 2 in, 2 out]
            n136 = property on="Motor" class="Clust (strict)"("Visible"=FALSE) -> ()  [unwired: 2 in, 2 out]
            n137 = property on="Rev/Fwd" class="Clust (strict)"("Visible"=FALSE) -> ()  [unwired: 2 in, 2 out]
            n138 = case shown="\"White Balance  **\"" w234 {
              tunnel: w233 -> [w240 w249 w258 w267 w276 _ w282]
              tunnel: w232 -> [w238 w246 w255 w264 w273 _ _]
              frame "Size  **" {
                n139 = Index Array(array=w238) -> (element=w237:cluster{string[]})  [unwired: 1 in]
                n140 = call <vilib>:"NT Read String.vi"("Name"=w240) -> ("String"=w239:string)  [unwired: 9 in, 1 out]
                n141 = Unbundle(w237) -> (w235:string[])
                n142 = Match First String(2:w235, 3:w239) -> (0:w236:i32)  [unwired: 1 out]
                n143 = property on="Test Ring" class="Ring (strict)"("Value"=w236, "Strings []"=w235) -> ()  [unwired: 2 in, 2 out]
                n144 = property on="Test Ring" class="Ring (strict)"("Visible"=TRUE) -> ()  [unwired: 2 in, 2 out]
                n145 = property on="Test Slider" class="Slide (strict)"("Visible"=FALSE) -> ()  [unwired: 2 in, 2 out]
              }
              frame "White Balance  **" {
                n146 = Index Array(array=w246, index=1) -> (element=w247:cluster{string[]})
                n147 = call <vilib>:"NT Read String.vi"("Name"=w249) -> ("String"=w248:string)  [unwired: 9 in, 1 out]
                n148 = Unbundle(w247) -> (w244:string[])
                n149 = Match First String(2:w244, 3:w248) -> (0:w243:i32)  [unwired: 1 out]
                n150 = property on="Test Ring" class="Ring (strict)"("Value"=w243, "Strings []"=w244) -> ()  [unwired: 2 in, 2 out]
                n151 = property on="Test Ring" class="Ring (strict)"("Visible"=TRUE) -> ()  [unwired: 2 in, 2 out]
                n152 = property on="Test Slider" class="Slide (strict)"("Visible"=FALSE) -> ()  [unwired: 2 in, 2 out]
              }
              frame "Exposure  **" {
                n153 = Index Array(array=w255, index=2) -> (element=w256:cluster{string[]})
                n154 = call <vilib>:"NT Read String.vi"("Name"=w258) -> ("String"=w257:string)  [unwired: 9 in, 1 out]
                n155 = Unbundle(w256) -> (w252:string[])
                n156 = Match First String(2:w252, 3:w257) -> (0:w253:i32)  [unwired: 1 out]
                n157 = property on="Test Ring" class="Ring (strict)"("Value"=w253, "Strings []"=w252) -> ()  [unwired: 2 in, 2 out]
                n158 = property on="Test Ring" class="Ring (strict)"("Visible"=TRUE) -> ()  [unwired: 2 in, 2 out]
                n159 = property on="Test Slider" class="Slide (strict)"("Visible"=FALSE) -> ()  [unwired: 2 in, 2 out]
              }
              frame "Exposure Priority  **" {
                n160 = Index Array(array=w264, index=3) -> (element=w265:cluster{string[]})
                n161 = call <vilib>:"NT Read String.vi"("Name"=w267) -> ("String"=w266:string)  [unwired: 9 in, 1 out]
                n162 = Unbundle(w265) -> (w261:string[])
                n163 = Match First String(2:w261, 3:w266) -> (0:w262:i32)  [unwired: 1 out]
                n164 = property on="Test Ring" class="Ring (strict)"("Value"=w262, "Strings []"=w261) -> ()  [unwired: 2 in, 2 out]
                n165 = property on="Test Ring" class="Ring (strict)"("Visible"=TRUE) -> ()  [unwired: 2 in, 2 out]
                n166 = property on="Test Slider" class="Slide (strict)"("Visible"=FALSE) -> ()  [unwired: 2 in, 2 out]
              }
              frame "Color Enable  **" {
                n167 = Index Array(array=w273, index=4) -> (element=w274:cluster{string[]})
                n168 = call <vilib>:"NT Read String.vi"("Name"=w276) -> ("String"=w275:string)  [unwired: 9 in, 1 out]
                n169 = Unbundle(w274) -> (w270:string[])
                n170 = Match First String(2:w270, 3:w275) -> (0:w271:i32)  [unwired: 1 out]
                n171 = property on="Test Ring" class="Ring (strict)"("Value"=w271, "Strings []"=w270) -> ()  [unwired: 2 in, 2 out]
                n172 = property on="Test Ring" class="Ring (strict)"("Visible"=TRUE) -> ()  [unwired: 2 in, 2 out]
                n173 = property on="Test Slider" class="Slide (strict)"("Visible"=FALSE) -> ()  [unwired: 2 in, 2 out]
              }
              frame Default {
                n174 = property on="Test Ring" class="Ring (strict)"("Visible"=FALSE) -> ()  [unwired: 2 in, 2 out]
                n175 = property on="Test Slider" class="Slide (strict)"("Visible"=FALSE) -> ()  [unwired: 2 in, 2 out]
              }
              frame "Brightness  **", "Color Level  **", "Compression  **", "FPS  **", "Sharpness  **" {
                n176 = call <vilib>:"NT Read Number.vi"("Name"=w282) -> ("Numeric"=w281:dbl)  [unwired: 9 in, 1 out]
                n177 = local write "Test Slider"(w281) -> ()
                n178 = property on="Test Slider" class="Slide (strict)"("Visible"=TRUE, "Scale.Maximum"=100.0 ("Scale.Range:Maximum")) -> ()  [unwired: 2 in, 2 out]
                n179 = property on="Test Ring" class="Ring (strict)"("Visible"=FALSE) -> ()  [unwired: 2 in, 2 out]
              }
            }
          }
        }
        n180 = property on="Progress" class="Clust (strict)"("Visible"=FALSE) -> ()  [unwired: 2 in, 2 out]
      }
      event "Test Name": Mouse Enter {
        # "Populate the ring with the list of tests"
        n181 = event-data() -> ()  [unwired: 1 in, 1 out]
        n182 = call <vilib>:"NT Read String Array.vi"("Name"="TestMode/TestList") -> ("String Array"=w290:string[])  [unwired: 9 in, 1 out]
        n183 = Build Array (concatenate)("Select the test to run...", w290) -> (w289:string[])
        n184 = property on="Test Name" class="Ring (strict)"("Strings []"=w289) -> ()  [unwired: 2 in, 2 out]
      }
      event "Test Name": Value Change {
        w292 = FALSE ("Visible")
        # "Tell the robot the test name to run"
        n185 = event-data() -> ("NewVal"=w296:u16)  [unwired: 1 in]
        n186 = property on="Test Name" class="Ring (strict)"() -> ("Strings []"=w297:string[])  [unwired: 2 in, 2 out]
        n187 = local write "Progress"(T8 {"Test Progress"=0, "Test Progress Text"=""} ("Progress")) -> ()
        n188 = Index Array(array=w297, index=w296) -> (element=w295:string)
        n189 = call <vilib>:"NT Write String.vi"("String"=w295, "Name"="TestMode/TestName") -> ()  [unwired: 9 in, 1 out]
        n190 = property on="Progress" class="Clust (strict)"("Visible"=TRUE) -> ()  [unwired: 2 in, 2 out]
        n191 = property on="Motor" class="Clust (strict)"("Visible"=w292) -> ()  [unwired: 2 in, 2 out]
        n192 = property on="Test Slider" class="Slide (strict)"("Visible"=w292) -> ()  [unwired: 2 in, 2 out]
        n193 = property on="On/Off" class="Bool (strict)"("Visible"=w292) -> ()  [unwired: 2 in, 2 out]
        n194 = property on="Rev/Fwd" class="Clust (strict)"("Visible"=w292) -> ()  [unwired: 2 in, 2 out]
        n195 = property on="Test Ring" class="Ring (strict)"("Visible"=w292) -> ()  [unwired: 2 in, 2 out]
      }
      event "Listbox": Double Click {
        # "Shift clears all"
        # "Update symbols on the listbox"
        n196 = event-data() -> ("PlatMods.Shift"=w300:bool, "Row"=w302:i32)  [unwired: 1 in]
        n197 = case shown="True" w300 {
          tunnel: w302 -> [w306 _]
          tunnel: 1 -> [w305 _]
          frame False {
            n198 = property on="Listbox" class="LstBox (strict)"() -> ("Item Symbols"=w304:i32[])  [unwired: 2 in, 2 out]
            n199 = Replace Array Subset(array=w304, new element=w305, index=w306) -> (w303:i32[])
            n200 = property on="Listbox" class="LstBox (strict)"("Item Symbols"=w303) -> ()  [unwired: 2 in, 2 out]
          }
          frame True {
            w307 = 0 ("Top Row")
            n201 = property on="Listbox" class="LstBox (strict)"() -> ("Number of Rows"=w309:u32)  [unwired: 2 in, 2 out]
            n202 = Initialize Array(0, w309) -> (w308:i32[])
            n203 = property on="Listbox" class="LstBox (strict)"("Top Row"=w307, "Value"=w307, "Item Symbols"=w308) -> ()  [unwired: 2 in, 2 out]
          }
        }
      }
      event "Listbox": Key Down {
        # "Update symbols on the listbox\nLeft and right keys check and uncheck"
        n204 = event-data() -> ("VKey"=w313:T21)  [unwired: 1 in]
        n205 = case shown="\"Left\", \"Right\"" w313 {
          selector: w313 -> [w318 _]
          tunnel: eventvkey."Left" ("VKey") -> [w316 _]
          frame "Left", "Right" {
            n206 = Equal?(x=w316, y=w318) -> (x = y?=w317:bool)
            n207 = Select(t=0, s=w317, f=1) -> (s? t:f=w319:i32)
            n208 = property on="Listbox" class="LstBox (strict)"() -> ("Item Symbols"=w322:i32[])  [unwired: 2 in, 2 out]
            n209 = Replace Array Subset(array=w322, new element=w319, index="Listbox") -> (w321:i32[])
            n210 = property on="Listbox" class="LstBox (strict)"("Item Symbols"=w321) -> ()  [unwired: 2 in, 2 out]
          }
          frame Default {
          }
        }
      }
      event "DB Camera Config": Value Change {
        # "Show or hide the cluster of controls, store in ini file"
        n211 = event-data() -> ("NewVal"=w326:bool)  [unwired: 1 in]
        n212 = case shown="False" w326 {
          tunnel: w325 -> [w335 _]
          tunnel: [w328 w346] -> w324
          tunnel: w323 -> [w327 w346]
          frame False {
            w342 = "Camera"
            w345 = FALSE ("Visible")
            n213 = local read "Camera Settings"() -> (w334:T3)
            n214 = Index Array(array=w335) -> (element=w338:cluster{string[]})  [unwired: 1 in]
            n215 = Unbundle(w334) -> ("Frame Rate"=w333:i32, "Compression"=w332:i32, "Size"=w336:u16)
            n216 = Unbundle(w338) -> (w337:string[])
            n217 = Index Array(array=w337, index=w336) -> (element=w331:string)
            n218 = call-poly <vilib>:"Write Key.vi"("section"=w342, "value"=w331, "key"="Size", "refnum"=w327) -> ("refnum out"=w344:T19)  [unwired: 2 in, 5 out]
            n219 = call-poly <vilib>:"Write Key.vi"("section"=w342, "value"=w333, "key"="FrameRate", "refnum"=w344) -> ("refnum out"=w343:T19)  [unwired: 1 in, 6 out]
            n220 = local write "DB Camera Config"(w345) -> ()
            n221 = property on="Camera Settings" class="Clust (strict)"("Visible"=w345) -> ()  [unwired: 2 in, 2 out]
            n222 = call-poly <vilib>:"Write Key.vi"("section"=w342, "value"=w332, "key"="Compression", "refnum"=w343) -> ("refnum out"=w329:T19)  [unwired: 1 in, 6 out]
            n223 = call <vilib>:"Close Config Data.vi"("refnum"=w329) -> ("file path"=w330:path)  [unwired: 2 in, 8 out]
            n224 = call <vilib>:"Open Config Data.vi"("configuration file path"=w330) -> ("refnum"=w328:T19)  [unwired: 8 in, 2 out]
          }
          frame True {
            n225 = property on="Camera Settings" class="Clust (strict)"("Visible"=TRUE) -> ()  [unwired: 2 in, 2 out]
          }
        }
      }
      event "Camera Settings": Value Change {
        # "Update summary string when any elements of DB camera change"
        n226 = event-data() -> ("NewVal"=w359:T3)  [unwired: 1 in]
        n227 = Index Array(array=w355) -> (element=w354:cluster{string[]})  [unwired: 1 in]
        n228 = Unbundle(w359) -> ("Frame Rate"=w350:i32, "Compression"=w349:i32, "Size"=w352:u16)
        n229 = Unbundle(w354) -> (w353:string[])
        n230 = Index Array(array=w353, index=w352) -> (element=w351:string)
        n231 = Format Into String(format string="%s   %dfps   %d%%", w351, w350, w349) -> (resulting string=w356:string)  [unwired: 2 in, 1 out]
        n232 = Build Array(w356) -> (w357:string[])
        n233 = property on="DB Camera Config" class="Bool (strict)"("Strings [4]"=w357) -> ()  [unwired: 2 in, 2 out]
      }
      event "Motor.Enable": Value Change {
        # "When the test mode otor enable helper is set, update that\ntree row item's value"
        n234 = event-data() -> ("NewVal"=w365:bool)  [unwired: 1 in]
        n235 = Unbundle("Motor") -> ("Value"=w364:dbl)  [unwired: 1 out]
        n236 = Select(t=w364, s=w365, f=0.0) -> (s? t:f=w362:dbl)
        n237 = call <vilib>:"NT Write Number.vi"("Numeric"=w362, "Name"=w361) -> ()  [unwired: 9 in, 1 out]
      }
      event "Test Slider": Value Change {
        # "When the test mode slider helper is set, update that\ntree row item's value"
        n238 = event-data() -> ("NewVal"=w368:dbl)  [unwired: 1 in]
        n239 = call <vilib>:"NT Write Number.vi"("Numeric"=w368, "Name"=w369) -> ()  [unwired: 9 in, 1 out]
      }
      event "On/Off": Value Change {
        # "When the test mode on/off helper value is set, update that\ntree row item's value"
        n240 = event-data() -> ("NewVal"=w373:bool)  [unwired: 1 in]
        n241 = Boolean To (0,1)(Boolean=w373) -> (0, 1=w372:i16)
        n242 = call <vilib>:"NT Write Number.vi"("Numeric"=w372, "Name"=w371) -> ()  [unwired: 9 in, 1 out]
      }
      event "Rev/Fwd": Value Change {
        # "When the test mode helper value for relays is set, update that\ntree row item's value"
        n243 = event-data() -> ("NewVal.Forward"=w381:bool, "NewVal.Reverse"=w380:bool)  [unwired: 1 in]
        n244 = Boolean To (0,1)(Boolean=w381) -> (0, 1=w377:i16)
        n245 = Boolean To (0,1)(Boolean=w380) -> (0, 1=w379:i16)
        n246 = Negate(x=w379) -> (-x=w378:i16)
        n247 = Add(x=w377, y=w378) -> (x+y=w376:i16)
        n248 = call <vilib>:"NT Write Number.vi"("Numeric"=w376, "Name"=w375) -> ()  [unwired: 9 in, 1 out]
      }
      event "Test Ring": Value Change {
        # "When a test mode helper value is selected from the ring,\nset the tree item's variable to the string value"
        n249 = event-data() -> ("NewVal"=w385:u16)  [unwired: 1 in]
        n250 = property on="Test Ring" class="Ring (strict)"() -> ("Strings []"=w386:string[])  [unwired: 2 in, 2 out]
        n251 = Index Array(array=w386, index=w385) -> (element=w384:string)
        n252 = call <vilib>:"NT Write String.vi"("String"=w384, "Name"=w383) -> ()  [unwired: 9 in, 1 out]
      }
      event "Rec Mode": Value Change {
        # "Update globals for recording mode and path to read log from.\nClear when logging and let NetworkTables set path for vision to\nuse."
        n253 = event-data() -> ("NewVal"=w396:enum32{"Stop", "Record", "Playback"})  [unwired: 1 in]
        n254 = global write "WPI_DashboardLogging Global.vi" "Logging Filename"(path "") -> ()
        n255 = global write "WPI_DashboardLogging Global.vi" "Recording"(w396) -> ()
        n256 = case shown="\"Playback\"" w396 {
          tunnel: w395 -> [_ w398 w406]
          tunnel: [_ _ w405] -> w392
          tunnel: [_ _ w404] -> _
          tunnel: w390 -> [_ _ w402]
          tunnel: cluster{i32, i32} {-250, 170} -> [_ _ w401]
          tunnel: [_ _ T22 {"Image Size"=TRUE, "Image Type"=TRUE, "Pixel Value"=TRUE, "ROI Information"=TRUE, "Zoom Factor"=FALSE} ("Image Information Shown:All Elements")] -> w388
          tunnel: [_ _ TRUE ("Zoom Factor")] -> w387
          frame Default {
          }
          frame "Stop", "Record" {
            # "Place Window too"
            n257 = invoke class="VI" method="FP.Close"(reference=w398) -> (reference out=w397:refnum<vi>)  [unwired: 2 in, 2 out]
            n258 = invoke class="VI" method="Abort VI"(reference=w397) -> ()  [unwired: 2 in, 3 out]
          }
          frame "Playback" {
            n259 = call "Open Playback Panel.vi"("Offset"=w401, "DB VI Ref"=w402, "Playback in"=w406) -> ("Playback out"=w403:refnum<vi>)  [unwired: 8 in]
            n260 = register-events(w403) -> (reference out=w405:refnum<event-registration>, error out=w404:errorcluster)  [unwired: 2 in]
          }
        }
        n261 = property on="Camera Image" class="ImageControl"("Image Information Shown"=w388, "Image Information Visible"=w387) -> ()  [unwired: 2 in, 2 out]
        n262 = call <vilib>:"WPI_DashboardNT Log FieldName Cache.vi"("Operation"=enum16{"Lookup/Add", "Index", "Clear"}."Clear") -> ()  [unwired: 8 in, 3 out]
      }
      event Panel Close {
        w407 = enum32{"Stop", "Record", "Playback"}."Stop" ("Rec Mode")
        # "Playback window has been closed, abort"
        n263 = event-data() -> ()  [unwired: 1 in, 4 out]
        n264 = local write "Rec Mode"(w407) -> ()
        n265 = global write "WPI_DashboardLogging Global.vi" "Recording"(w407) -> ()
      }
      event Panel Close {
        # "Abort playback window and ourself"
        n266 = event-data() -> ()  [unwired: 1 in, 4 out]
        n267 = invoke class="VI" method="FP.Close"(reference=w412) -> (reference out=w411:refnum<vi>)  [unwired: 2 in, 2 out]
        n268 = invoke class="VI" method="Abort VI"(reference=w411) -> (error out=w410:errorcluster)  [unwired: 2 in, 2 out]
        n269 = invoke class="VI" method="Abort VI"(error in=w410) -> ()  [unwired: 2 in, 3 out]
      }
      event "Vision": Value Change {
        # "Enable/Disable Compression slider.\nHW USB is hard-coded into the camera"
        n270 = event-data() -> ("NewVal"=w418:u16)  [unwired: 1 in]
        n271 = Equal?(x=w418, y=u32 2 ("milliseconds to wait")) -> (x = y?=w416:bool)
        n272 = Select(t=T23."Disabled and Grayed Out" ("Disabled"), s=w416, f=T23."Enabled" ("Disabled")) -> (s? t:f=w413:T23)
        n273 = property on="Compression" class="Slide (strict)"("DisabledEnum"=w413) -> ()  [unwired: 2 in, 2 out]
      }
    }
  }
  n274 = while {
    tunnel: w38 -> [w421]
    i -> [w424]
    stop <- FALSE stop-if-true
    n275 = Wait (ms)(milliseconds to wait=u32 100) -> ()  [unwired: 1 out]
    n276 = case shown="\"Playback\"" "Rec Mode" {
      tunnel: w424 -> [_ _ w439]
      tunnel: [u32 2829099 ("Base Color") u32 11141120 ("Target Color") w428] -> w420
      frame "Stop", Default {
        # "Reset the color, extra updates don't cost much"
      }
      frame "Record" {
      }
      frame "Playback" {
        # "Playback"
        n277 = Quotient & Remainder(x=w439, y=u32 50 ("milliseconds to wait")) -> (x-y*floor(x/y)=w435:u32)  [unwired: 1 out]
        n278 = Divide(x=w435, y=u32 50 ("milliseconds to wait")) -> (x/y=w432:dbl)
        n279 = Multiply(x=6.283185307179586, y=w432) -> (x*y=w437:dbl)
        n280 = Sine(x=w437) -> (sin(x)=w436:dbl)
        n281 = Absolute Value(x=w436) -> (abs(x)=w429:dbl)
        n282 = call "Interpolate RGB Color.vi"("Proportion"=w429, "Target Color"=u32 30976, "Base Color"=u32 2829099) -> ("Result Color"=w428:u32)  [unwired: 8 in]
      }
    }
    n283 = property class="Pane"(reference=w421, "PaneColor"=w420) -> ()  [unwired: 1 in, 2 out]
  }
  n284 = TCP Create Listener(10:u16 1741 ("timeout ms (25000)")) -> (3:w1:refnum<k5>)  [unwired: 4 in, 2 out]
  n285 = while {
    tunnel: w1 -> [w441]
    stop <- FALSE stop-if-true
    n286 = TCP Wait On Listener(11:w441) -> (4:w440:refnum<k5>)  [unwired: 3 in, 4 out]
    n287 = local write "TCP"(w440) -> ()
  }
  n288 = property on="On/Off" class="Bool (strict)"("Visible"=w6) -> ()  [unwired: 2 in, 2 out]
  n289 = property on="Motor" class="Clust (strict)"("Visible"=w6) -> ()  [unwired: 2 in, 2 out]
  n290 = property on="Progress" class="Clust (strict)"("Visible"=w6) -> ()  [unwired: 2 in, 2 out]
  n291 = property on="Test Ring" class="Ring (strict)"("Visible"=w6) -> ()  [unwired: 2 in, 2 out]
  n292 = property on="Rev/Fwd" class="Clust (strict)"("Visible"=w6) -> ()  [unwired: 2 in, 2 out]
  n293 = local write "DB Camera Config"(w6) -> ()
  n294 = property on="Camera Settings" class="Clust (strict)"("Visible"=w6) -> ()  [unwired: 2 in, 2 out]
  n295 = global write "WPI_DashboardLogging Global.vi" "Recording"(w32) -> ()
  n296 = local write "Rec Mode"(w32) -> ()
